vi "tcsOfc_acceptCommand_readShwfsFile.vi"(8 "error in (no error)":errorcluster, 11 "command_readShwfsFile_Ctl":T1) -> (0 "error out":errorcluster, 2 "function return":i32, 3 "command_readShwfsFile_Ctl out":T1)   [LabVIEW 2016, in "SALLV_tcsOfc.lvlib"]
doc: "int tcsOfc_shm_acceptCommand_readShwfsFileLV(tcsOfc_command_readShwfsFileLV *command_readShwfsFile_Ctl );"
uses:
  SALLV_tcsOfc.lvlib
  DataTypes/command_readShwfsFile.ctl
  SALLV_tcsOfc.so
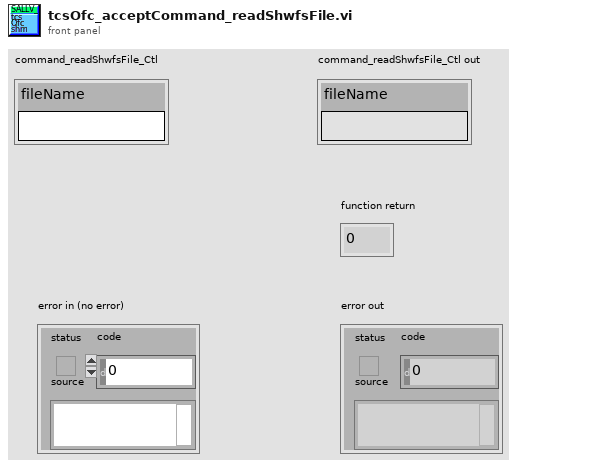
[diagram p1: front panel]
types:
  T1 = typedef "SALLV_tcsOfc.lvlib/command_readShwfsFile.ctl" = cluster{"fileName":string}
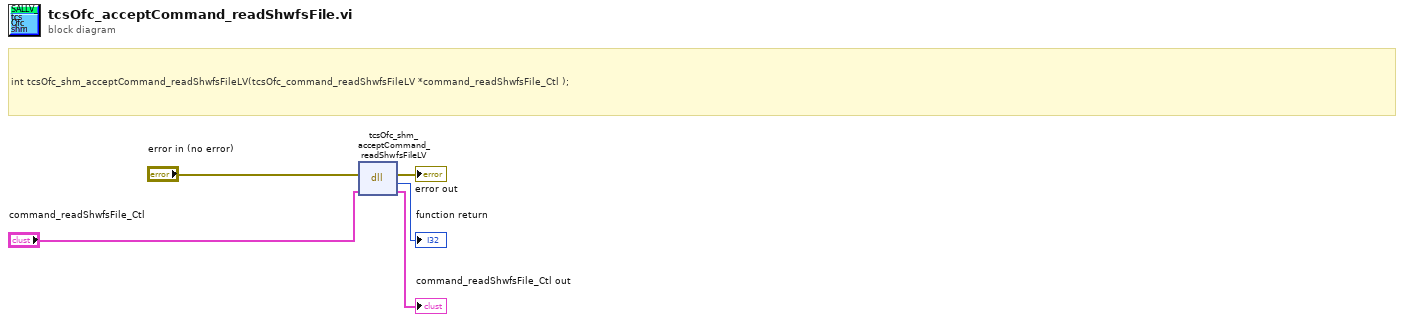
[diagram p0: block diagram]
diagram:
  # "int tcsOfc_shm_acceptCommand_readShwfsFileLV(tcsOfc_command_readShwfsFileLV *command_readShwfsFile_Ctl );"
  n1 = dll-call lib="home/ttsai/Documents/salAPI/SALLV_tcsOfc/SALLV_tcsOfc.*" fn="tcsOfc_shm_acceptCommand_readShwfsFileLV"(error in="error in (no error)", "command_readShwfsFile_Ctl"="command_readShwfsFile_Ctl") -> (error out=→"error out":errorcluster, →"function return":i32, "command_readShwfsFile_Ctl"=→"command_readShwfsFile_Ctl out":T1)  [unwired: 2 in, 1 out]
